vi "CalculateCurvature.vi"(9 "Lookahead":dbl, 10 "Point":cluster{"x":dbl, "y":dbl}, 11 "Robot":T1 {"Angle" scale=0.0..360.0; "Point"."y" scale=-10.0..10.0; "Point"."x" scale=-10.0..10.0}) -> (3 "Curvature":dbl)   [LabVIEW 2016]
panel:
  out "output variable":dbl
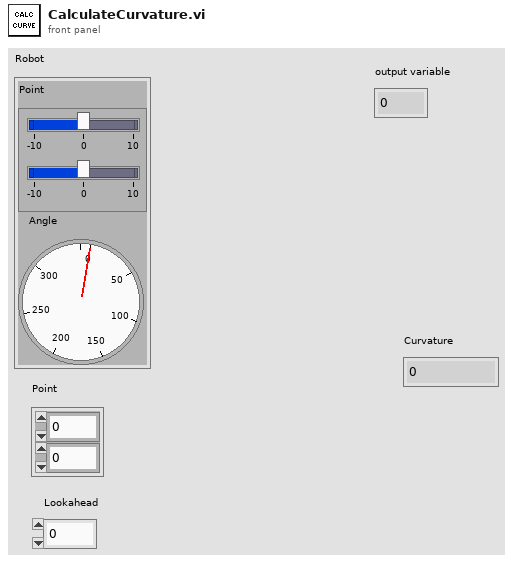
[diagram p1: front panel]
types:
  T1 = cluster{"Point":cluster{"x":dbl, "y":dbl}, "Angle":dbl}
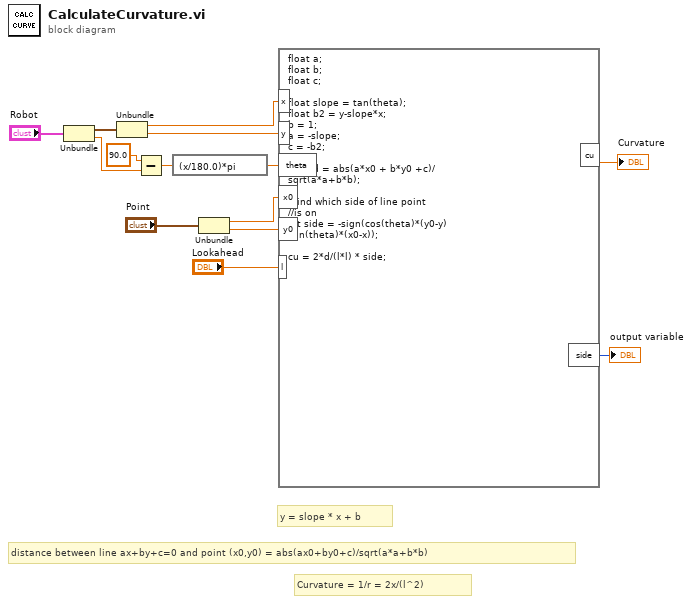
[diagram p0: block diagram]
diagram:
  # "Curvature = 1/r = 2x/(l^2)"
  # "y = slope * x + b"
  # "distance between line ax+by+c=0 and point (x0,y0) = abs(ax0+by0+c)/sqrt(a*a+b*b)"
  n1 = Unbundle("Robot") -> ("Point"=w13:cluster{"x":dbl, "y":dbl}, "Angle"=w3:dbl)
  n2 = Unbundle(w13) -> ("x"=w12:dbl, "y"=w11:dbl)
  n3 = Subtract(x=90.0, y=w3) -> (x-y=w2:dbl)
  n4 = expression code="(x/180.0)*pi" ("degrees to radians")(w2) -> (w10:dbl)
  n5 = Unbundle("Point") -> ("x"=w8:dbl, "y"=w7:dbl)
  n6 = formula code="float a;\nfloat b;\nfloat c;\n\nfloat slope = tan(theta);\nfloat b2 = y-slope*x;\nb = 1;\na = -slope;\nc = -b2;\n\nfloat d = abs(a*x0 + b*y0 +c)/\nsqrt(a*a+b*b);\n\n//find which side of line point\n//is on\nint side = -sign(cos(theta)*(y0-y)\n-sin(theta)*(x0-x));\n\ncu = 2*d/(l*l) * side;"("x"=w12, "y"=w11, "theta"=w10, "x0"=w8, "y0"=w7, "l"="Lookahead") -> ("cu"=→"Curvature":dbl, "side"=→"output variable":i32)
